vi "Waterfall Plot.vi"(6 "averaging parameters":T1={"averaging mode"=enum."No averaging", "weighting mode"=enum."Exponential", "number of averages"=10} {"number of averages" min=1}, 8 "window":T2=1 items=["Rectangle"=0, "Hanning"=1, "Hamming"=2, "Blackman-Harris"=3, "Exact Blackman"=4, "Blackman"=5, "Flat Top"=6, "4 Term B-Harris "=7, "7 Term B-Harris"=8, "Low Sidelobe"=9, "Blackman Nuttall"=11, "Triangle"=30, "Bartlett-Hanning"=31, "Bohman"=32, "Parzen"=33, "Welch"=34, "Kaiser"=60, "Dolph-Chebyshev"=61, "Gaussian"=62], 9 "Slice":dbl, 10 "Channel Name in":string, 11 "Signal":waveform(dbl)={"t0"=timestamp(0 s since 1904-01-01), "dt"=0.0, "Y"=[]}) -> ()   [LabVIEW 2024, in "Waterfall.lvlib" / "Waterfall.lvclass"]
uses:
  Waterfall.lvclass
  <vilib>/Math Plots/3D Math Plots/3D Waterfall/3D Waterfall XCtrl/3D Waterfall.xctl
  <vilib>/Analysis/4window.llb/windowTd.ctl
  <vilib>/Waveform/WDTOps.llb/WDT Waveform Duration DBL.vi
  <vilib>/Waveform/WDTOps.llb/WDT Get Waveform Subset DBL.vi
  <vilib>/measure/maspectr.llb/FFT Power Spectrum and PSD for 1 Chan.vi
  <vilib>/Math Plots/3D Math Plots/3D Waterfall/3D Waterfall Datatype/Public/Plot Helper (Vector).vi
  Waterfall.lvclass/Waterfall.ctl
  <vilib>/Math Plots/3D Math Plots/3D Waterfall/3D Waterfall Datatype/3D Waterfall Datatype.lvclass
  <vilib>/measure/NI_MAPro.lvlib
  <vilib>/Analysis/NI_AALPro.lvlib
panel:
  out "Time Domain 3D Waterfall":refnum<class "3D Plot Datatype.lvclass">[](xcontrol)
  out "Frequency Domain 3D Waterfall":refnum<class "3D Plot Datatype.lvclass">[](xcontrol)
  out "Channel Name":string
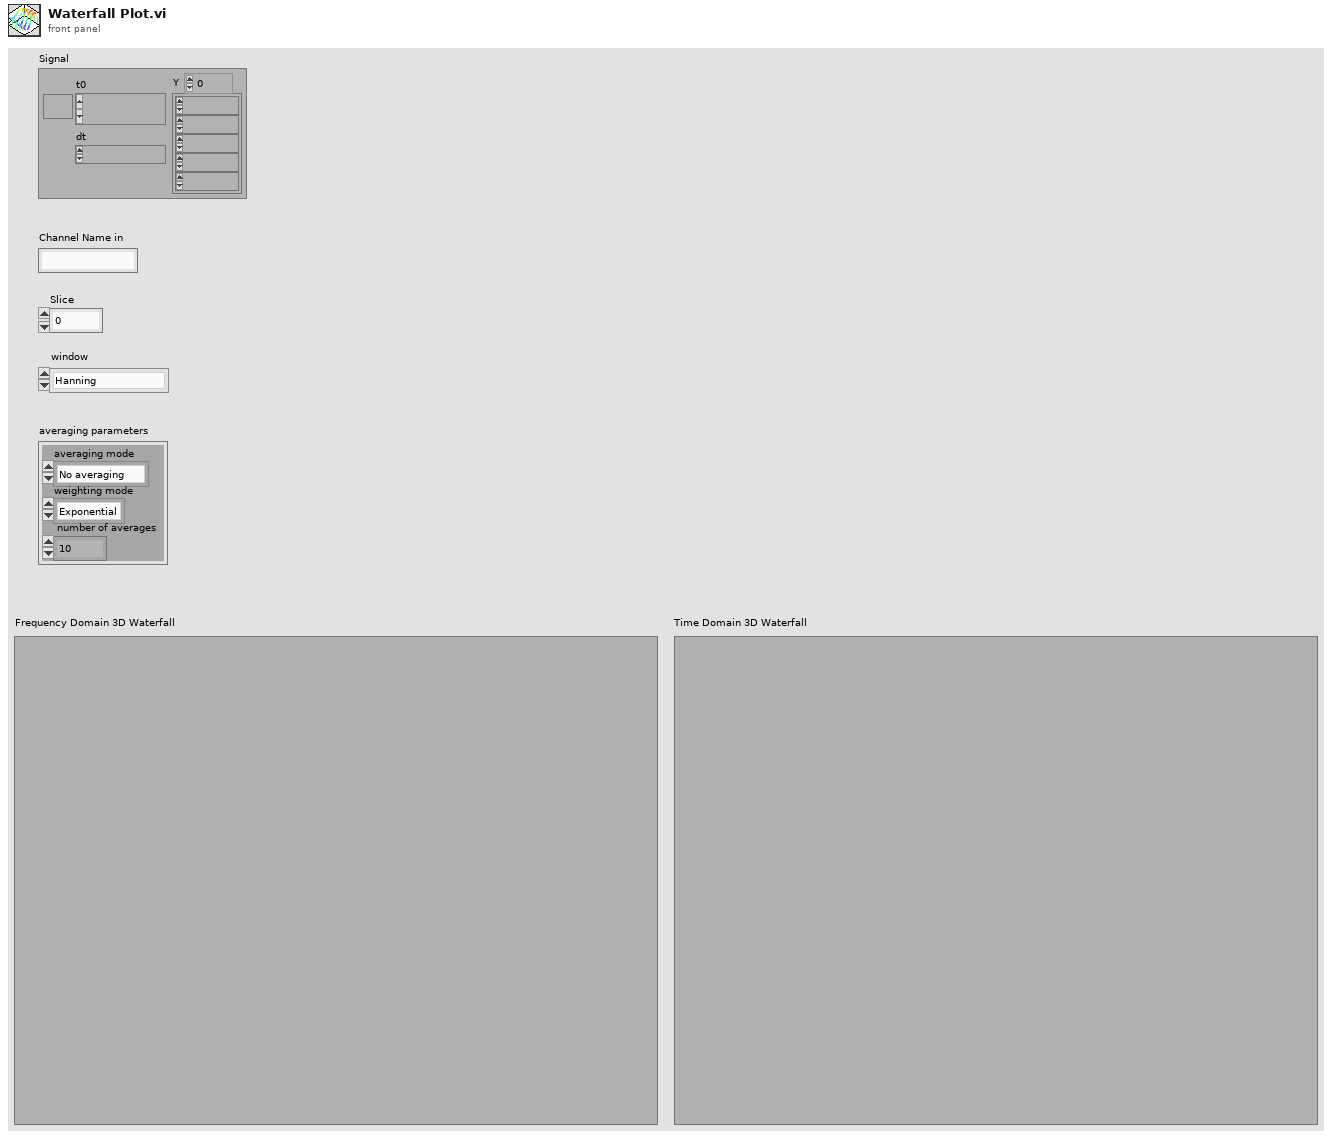
[diagram p1: front panel]
types:
  T1 = cluster{"averaging mode":enum16{"No averaging", "Vector averaging", "RMS averaging", "Peak hold"}, "weighting mode":enum16{"Linear", "Exponential"}, "number of averages":u32}
  T2 = typedef "NI_AALPro.lvlib/windowTd.ctl" = u32
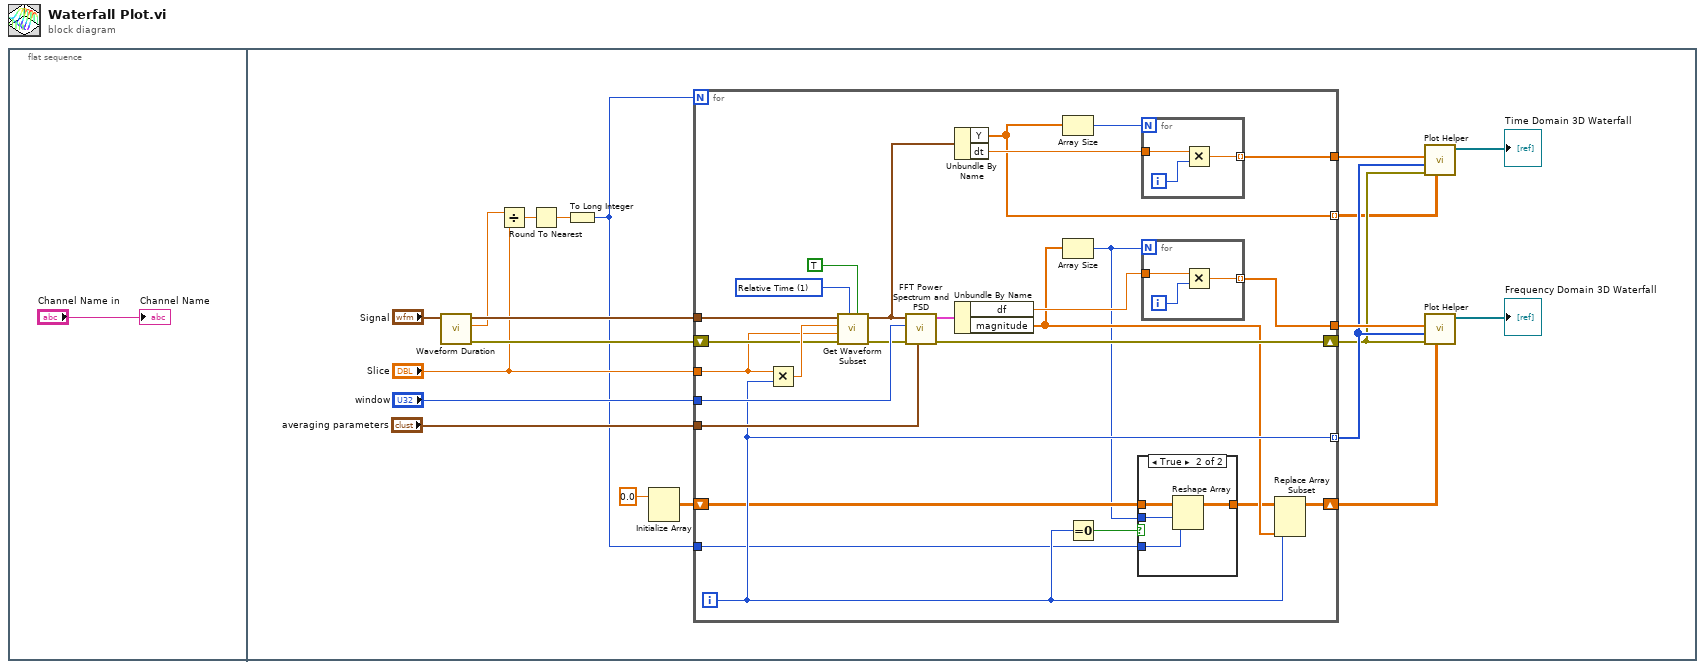
[diagram p0: block diagram]
diagram:
  n1 = flat-sequence {
    frame #0 {
      "Channel Name" <- "Channel Name in"
    }
    frame #1 {
      n2 = call-poly <vilib>:"Waveform Duration.vi"("waveform in"="Signal") -> ("error out"=w19:errorcluster, "duration"=w8:dbl, "waveform out"=w20:waveform(dbl))  [unwired: 8 in]
      n3 = Divide(x=w8, y="Slice") -> (x/y=w21:dbl)
      n4 = Round To Nearest(number=w21) -> (nearest integer value=w10:dbl)
      n5 = To Long Integer(number=w10) -> (32bit integer=w9:i32)
      n6 = Initialize Array(0.0 ("element")) -> (w16:dbl[][])  [unwired: 2 in]
      n7 = for {
        N: w9 -> [_]
        tunnel: w20 -> [w47]
        tunnel: "Slice" -> [w35]
        tunnel: [w41] -> w17
        shift-right: [w40] -> w5
        shift-left: w19 -> [w43]
        tunnel: [w34] -> w6 mode=indexing
        shift-right: [w39] -> w14
        shift-left: w16 -> [w31]
        tunnel: "window" -> [w38]
        tunnel: "averaging parameters" -> [w37]
        tunnel: w9 -> [w30]
        tunnel: [w24] -> w3 mode=indexing
        tunnel: [w25] -> w4
        i -> [w34]
        w45 = u16 1 items=["Samples", "Relative Time"] ("start/duration format")
        n8 = Multiply(x=w35, y=w34) -> (x*y=w46:dbl)
        n9 = call-poly <vilib>:"Get Waveform Subset.vi"("open interval? (T)"=TRUE, "start/duration format"=w45, "error in (no error)"=w43, "duration"=w35, "start samples/time"=w46, "waveform in"=w47) -> ("error out"=w22:errorcluster, "waveform out"=w23:waveform(dbl))  [unwired: 2 out]
        n10 = call-poly <vilib>:"FFT Power Spectrum and PSD.vi"("averaging parameters"=w37, "error in (no error)"=w22, "window"=w38, "time signal"=w23) -> ("error out"=w40:errorcluster, "Power Spectrum / PSD"=w42:cluster{"f0":dbl, "df":dbl, "magnitude":dbl[]})  [unwired: 4 in, 2 out]
        n11 = Unbundle By Name(w23) -> ("Y"=w24:dbl[], "dt"=w28:dbl)
        n12 = Unbundle By Name(w42) -> ("df"=w36:dbl, "magnitude"=w32:dbl[])
        n13 = Array Size(array=w24) -> (size(s)=w26:i32)
        n14 = Array Size(array=w32) -> (size(s)=w27:i32)
        n15 = Equal To 0?(x=w34) -> (x = 0?=w33:bool)
        n16 = case shown="True" w33 {
          tunnel: w31 -> [w51 w55]
          tunnel: w30 -> [_ w54]
          tunnel: w27 -> [_ w53]
          tunnel: [w51 w52] -> w29
          frame False {
          }
          frame True {
            n17 = Reshape Array(w55, w53, w54) -> (w52:dbl[][])
          }
        }
        n18 = for {
          N: w26 -> [_]
          tunnel: w28 -> [w50]
          tunnel: [w49] -> w25 mode=indexing
          i -> [w48]
          n19 = Multiply(x=w50, y=w48) -> (x*y=w49:dbl)
        }
        n20 = for {
          N: w27 -> [_]
          tunnel: w36 -> [w58]
          tunnel: [w57] -> w41 mode=indexing
          i -> [w56]
          n21 = Multiply(x=w58, y=w56) -> (x*y=w57:dbl)
        }
        n22 = Replace Array Subset(array=w29, new element=w32, index (col)=w34) -> (w39:dbl[][])  [unwired: 1 in]
      }
      n23 = call-poly <vilib>:"Plot Helper.vi"("z matrix"=w3, "error in (no error)"=w5, "y vector"=w6, "x vector"=w4) -> ("3D Plot lvclass Array out"=→"Time Domain 3D Waterfall":refnum<class "3D Plot Datatype.lvclass">[])  [unwired: 2 in, 5 out]
      n24 = call-poly <vilib>:"Plot Helper.vi"("z matrix"=w14, "error in (no error)"=w5, "y vector"=w6, "x vector"=w17) -> ("3D Plot lvclass Array out"=→"Frequency Domain 3D Waterfall":refnum<class "3D Plot Datatype.lvclass">[])  [unwired: 2 in, 5 out]
    }
  }
